vi "Zufallszahl zwischen 1 und.vi"(1 "Zufallszahl \nzwischen 1 und":dbl) -> (0 "Zufallszahl":dbl)   [LabVIEW 2014]
panel:
  out "nearest integer value 2":dbl
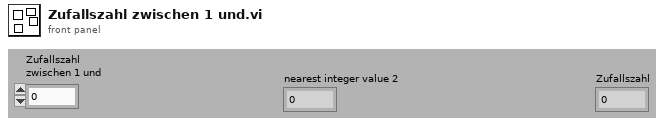
[diagram p1: front panel]
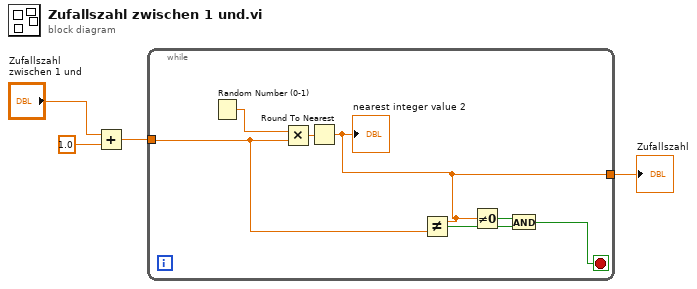
[diagram p0: block diagram]
diagram:
  n1 = Add(x="Zufallszahl \nzwischen 1 und", y=1.0) -> (x+y=w1:dbl)
  n2 = while {
    tunnel: w1 -> [w9]
    tunnel: [w5] -> w4
    stop <- w6 stop-if-true
    n3 = Random Number (0-1)() -> (number: 0 to 1=w10:dbl)
    n4 = Multiply(x=w10, y=w9) -> (x*y=w11:dbl)
    n5 = Round To Nearest(number=w11) -> (nearest integer value=w5:dbl)
    "nearest integer value 2" <- w5
    n6 = Not Equal?(x=w5, y=w9) -> (x != y?=w7:bool)
    n7 = Not Equal To 0?(x=w5) -> (x != 0?=w8:bool)
    n8 = And(x=w8, y=w7) -> (x .and. y?=w6:bool)
  }
  "Zufallszahl" <- w4
